vi "dfd_Get Linear Phase Factors.vi"(8 "error in (no error)":errorcluster, 9 "gain":dbl, 10 "zeros":cdb[](array[numeric])) -> (0 "error out":errorcluster, 2 "H(n) 2":dbl[](array[numeric]), 3 "H(n) 1":dbl[](array[numeric]))   [LabVIEW 2017, in "NI_DigFilter_Design.lvlib"]
doc: "Performs linear phase spectral factorization according to the filter's zeros."
uses:
  <vilib>/addons/Digital Filter Design/NI_DigFilter_Design.lvlib
  <vilib>/addons/Digital Filter Design/_Misc.llb/dfd_Error Cluster From Error Code (Array).vi
  <vilib>/Analysis/polynomials.llb/Create Polynomial From Roots (CDB).vi
  <vilib>/addons/Digital Filter Design/StructCvt.llb/dfd_Get Alternate Components of Array (Complex).vi
  <vilib>/Analysis/NI_AALPro.lvlib
  <vilib>/addons/Digital Filter Design/NI_DigFilterLicensed.lvlib
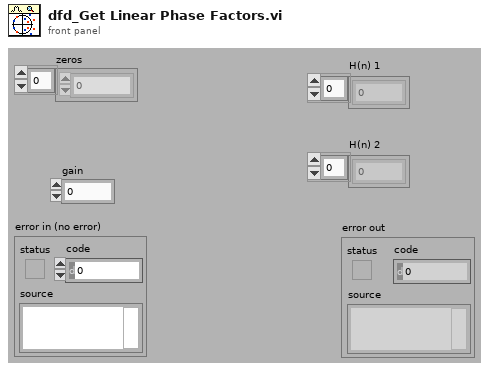
[diagram p1: front panel]
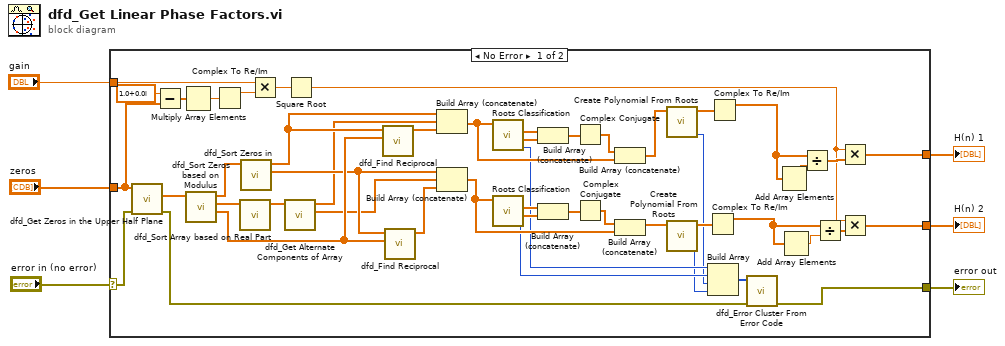
[diagram p0: block diagram]
diagram:
  n1 = case shown="No Error" "error in (no error)" {
    selector: "error in (no error)" -> [w31 w56]
    tunnel: [w8 _] -> w6
    tunnel: [w7 _] -> w5
    tunnel: [w11 w56] -> w4
    tunnel: "zeros" -> [w24 _]
    tunnel: "gain" -> [w20 _]
    frame No Error {
      n2 = call <vilib>:"dfd_Get Zeros in the Upper Half Plane.vi"("error in (no error)"=w31, "zeros"=w24) -> ("error out"=w32:errorcluster, "half zeros"=w47:cdb[])  [unwired: 2 in, 6 out]
      n3 = Subtract(x=cdb 1.0+0.0i, y=w24) -> (x-y=w23:cdb[])
      n4 = Multiply Array Elements(1:w23) -> (0:w22:cdb)
      n5 = call <vilib>:"dfd_Sort Zeros based on Modulus.vi"("zeros"=w47) -> (">1"=w43:cdb[], "=1"=w46:cdb[], "<1"=w39:cdb[])  [unwired: 8 out]
      n6 = Complex To Re/Im(x + iy=w22) -> (x=w19:dbl)  [unwired: 1 out]
      n7 = call <vilib>:"dfd_Sort Array based on Real Part.vi"("input array"=w46) -> ("sorted array"=w45:cdb[])  [unwired: 10 out]
      n8 = call <vilib>:"dfd_Sort Zeros in.vi"("zeros in"=w39) -> ("another half"=w37:cdb[], "half zeros"=w38:cdb[])  [unwired: 9 out]
      n9 = Multiply(x=w20, y=w19) -> (x*y=w21:dbl)
      n10 = call-poly <vilib>:"dfd_Get Alternate Components of Array.vi"("input array"=w45) -> ("another half"=w36:cdb[], "half array"=w35:cdb[])  [unwired: 9 out]
      n11 = Square Root(x=w21) -> (sqrt(x)=w26:dbl)
      n12 = call <vilib>:"dfd_Find Reciprocal.vi"("zeros out"=w43, "zeros in"=w38) -> ("reciprocal"=w42:cdb[])  [unwired: 9 out]
      n13 = call <vilib>:"dfd_Find Reciprocal.vi"("zeros out"=w43, "zeros in"=w37) -> ("reciprocal"=w44:cdb[])  [unwired: 9 out]
      n14 = Build Array (concatenate)(w38, w35, w42) -> (w41:cdb[])
      n15 = Build Array (concatenate)(w37, w36, w44) -> (w40:cdb[])
      n16 = call <vilib>:"Roots Classification.vi"("Roots"=w41) -> ("error"=w34:i32, "Pure Complex Roots"=w50:cdb[], "Complex Pair Roots"=w49:cdb[])  [unwired: 2 in, 6 out]
      n17 = call <vilib>:"Roots Classification.vi"("Roots"=w40) -> ("error"=w33:i32, "Pure Complex Roots"=w54:cdb[], "Complex Pair Roots"=w55:cdb[])  [unwired: 2 in, 6 out]
      n18 = Build Array (concatenate)(w49, w50) -> (w51:cdb[])
      n19 = Build Array (concatenate)(w55, w54) -> (w53:cdb[])
      n20 = Complex Conjugate(1:w51) -> (0:w48:cdb[])
      n21 = Complex Conjugate(1:w53) -> (0:w52:cdb[])
      n22 = Build Array (concatenate)(w48, w41) -> (w18:cdb[])
      n23 = Build Array (concatenate)(w52, w40) -> (w16:cdb[])
      n24 = call-poly <vilib>:"Create Polynomial From Roots.vi"("Roots"=w18) -> ("error"=w14:i32, "P(x)"=w17:cdb[])  [unwired: 9 out]
      n25 = call-poly <vilib>:"Create Polynomial From Roots.vi"("Roots"=w16) -> ("error"=w13:i32, "P(x)"=w15:cdb[])  [unwired: 9 out]
      n26 = Complex To Re/Im(x + iy=w15) -> (x=w9:dbl[])  [unwired: 1 out]
      n27 = Build Array(w34, w33, w14, w13) -> (w12:i32[])
      n28 = Complex To Re/Im(x + iy=w17) -> (x=w10:dbl[])  [unwired: 1 out]
      n29 = call-poly <vilib>:"dfd_Error Cluster From Error Code.vi"("error in (no error)"=w32, "error code (0)"=w12) -> ("error out"=w11:errorcluster)  [unwired: 9 out]
      n30 = Add Array Elements(numeric array=w10) -> (sum=w29:dbl)
      n31 = Add Array Elements(numeric array=w9) -> (sum=w28:dbl)
      n32 = Divide(x=w10, y=w29) -> (x/y=w30:dbl[])
      n33 = Divide(x=w9, y=w28) -> (x/y=w27:dbl[])
      n34 = Multiply(x=w26, y=w30) -> (x*y=w7:dbl[])
      n35 = Multiply(x=w26, y=w27) -> (x*y=w8:dbl[])
    }
    frame Error {
    }
  }
  "H(n) 2" <- w6
  "H(n) 1" <- w5
  "error out" <- w4
